vi "InstrumentsTree.vi"(1 "Type":string) -> (0 "Name":string)   [LabVIEW 2009]
uses:
  <userlib>/_OpenG.lib/array/array.llb/Conditional Auto-Indexing Tunnel (String)__ogtk.vi
panel:
  in  "Tree":string(tree)
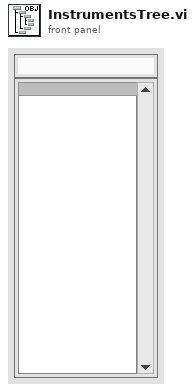
[diagram p1: front panel]
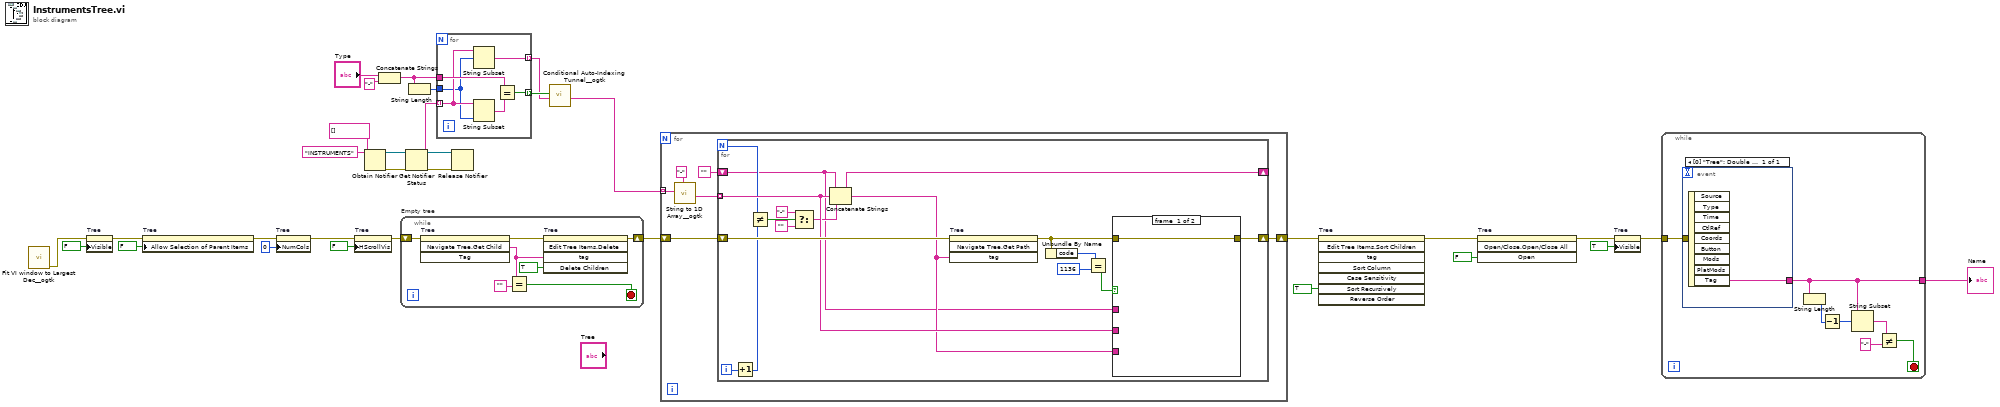
[diagram p0: block diagram]
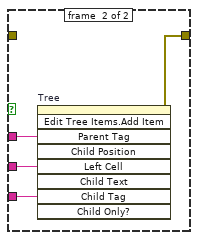
[diagram p2: hidden frame]
diagram:
  n1 = call <userlib>:"Fit VI window to Largest Dec__ogtk.vi"() -> ("error out"=w1:errorcluster)  [unwired: 3 in, 4 out]
  n2 = property on="Tree" class="Tree (strict)"(error in=w1, "Visible"=FALSE) -> (error out=w23:errorcluster)  [unwired: 1 in, 1 out]
  n3 = property on="Tree" class="Tree (strict)"(error in=w23, "Allow Selection of Parent Items"=FALSE) -> (error out=w28:errorcluster)  [unwired: 1 in, 1 out]
  n4 = property on="Tree" class="Tree (strict)"(error in=w28, "NumCols"=u32 0 ("Number of Columns")) -> (error out=w25:errorcluster)  [unwired: 1 in, 1 out]
  n5 = property on="Tree" class="Tree (strict)"(error in=w25, "HScrollVis"=FALSE ("Visible Items:Horizontal Scrollbar Visible")) -> (error out=w24:errorcluster)  [unwired: 1 in, 1 out]
  n6 = Obtain Notifier(name (unnamed)="INSTRUMENTS", notification data type=string[] [] ("Motor Names")) -> (notifier out=w13:refnum<notifier>, error out=w12:errorcluster)  [unwired: 2 in, 1 out]
  n7 = Concatenate Strings("Type", "-" ("string")) -> (w6:string)
  n8 = while "Empty tree" {
    shift-right: [w34] -> w32
    shift-left: w24 -> [w33]
    stop <- w36 stop-if-true
    n9 = invoke on="Tree" class="Tree (strict)" method="Navigate Tree.Get Child"(error in=w33) -> (error out=w35:errorcluster, "Navigate Tree:Get Child"=w38:string)  [unwired: 3 in, 2 out]
    n10 = Equal?(x=w38, y="") -> (x = y?=w36:bool)
    n11 = invoke on="Tree" class="Tree (strict)" method="Edit Tree Items.Delete"(error in=w35, "tag"=w38, "Delete Children"=TRUE ("Delete Children?")) -> (error out=w34:errorcluster)  [unwired: 2 in, 4 out]
  }
  n12 = Get Notifier Status(notifier=w13, error in (no error)=w12) -> (notifier out=w10:refnum<notifier>, current notification=w4:string[], error out=w11:errorcluster)  [unwired: 2 out]
  n13 = String Length(string=w6) -> (length=w9:i32)
  n14 = for {
    tunnel: w4 -> [w42] mode=indexing
    tunnel: w6 -> [w45]
    tunnel: w9 -> [w41]
    tunnel: [w43] -> w5 mode=indexing
    tunnel: [w40] -> w3 mode=indexing
    n15 = String Subset(string=w42, offset (0)=w41) -> (substring=w40:string)  [unwired: 1 out]
    n16 = String Subset(string=w42, length (rest)=w41) -> (substring=w44:string)  [unwired: 1 out]
    n17 = Equal?(x=w45, y=w44) -> (x = y?=w43:bool)
  }
  n18 = Release Notifier(notifier=w10, error in (no error)=w11) -> ()  [unwired: 4 out]
  n19 = call-poly <userlib>:"Conditional Auto-Indexing Tunnel__ogtk.vi"("Array in"=w3, "Elements to keep"=w5) -> ("Filtered Array out"=w2:string[])  [unwired: 5 out]
  n20 = for {
    tunnel: w2 -> [w48] mode=indexing
    shift-right: [w50] -> w31
    shift-left: w32 -> [w47]
    n21 = call <userlib>:"String to 1D Array__ogtk.vi"("delimiter (Tab)"="-", "string"=w48) -> ("Array of Strings"=w49:string[])  [unwired: 1 in, 8 out]
    n22 = for {
      N -> [w59]
      tunnel: w49 -> [w64] mode=indexing
      shift-right: [w63] -> w50
      shift-left: w47 -> [w67]
      shift-right: [w53] -> _
      shift-left: "" -> [w52]
      i -> [w60]
      n23 = Increment(x=w60) -> (x+1=w58:i32)
      n24 = Not Equal?(x=w59, y=w58) -> (x != y?=w57:bool)
      n25 = Select(t="-", s=w57, f="") -> (s? t:f=w54:string)
      n26 = Concatenate Strings(w52, w64, w54) -> (w53:string)
      n27 = invoke on="Tree" class="Tree (strict)" method="Navigate Tree.Get Path"(error in=w67, "tag"=w53) -> (error out=w61:errorcluster)  [unwired: 2 in, 3 out]
      n28 = Unbundle By Name(w61) -> ("code"=w66:i32)
      n29 = Equal?(x=w66, y=1136) -> (x = y?=w62:bool)
      n30 = case shown="True" w62 {
        tunnel: w64 -> [_ w72]
        tunnel: w53 -> [_ w71]
        tunnel: [w68 w70] -> w63
        tunnel: w61 -> [w68 _]
        tunnel: w52 -> [_ w69]
        frame #0 {
        }
        frame #1 {
          n31 = invoke on="Tree" class="Tree (strict)" method="Edit Tree Items.Add Item"("Parent Tag"=w69, "Left Cell"=w72, "Child Tag"=w71) -> (error out=w70:errorcluster)  [unwired: 6 in, 8 out]
        }
      }
    }
  }
  n32 = invoke on="Tree" class="Tree (strict)" method="Edit Tree Items.Sort Children"(error in=w31, "Sort Recursively"=TRUE ("Sort Recursively?")) -> (error out=w18:errorcluster)  [unwired: 6 in, 7 out]
  n33 = invoke on="Tree" class="Tree (strict)" method="Open/Close.Open/Close All"(error in=w18, "Open"=FALSE ("Open?")) -> (error out=w17:errorcluster)  [unwired: 2 in, 3 out]
  n34 = property on="Tree" class="Tree (strict)"(error in=w17, "Visible"=TRUE) -> (error out=w20:errorcluster)  [unwired: 1 in, 1 out]
  n35 = while {
    tunnel: w20 -> [w79]
    tunnel: [w78] -> w19
    stop <- w73 stop-if-true
    n36 = event shown="[0] \"Tree\": Double Click" {
      selector: _ -> [_]
      dyn-events: _ -> [_]
      timeout: _ -> [_]
      tunnel: w79 -> [_]
      tunnel: [w80] -> w78
      event [0] "Tree": Double Click {
        n37 = event-data() -> ("Tag"=w80:string)  [unwired: 9 out]
      }
    }
    n38 = String Length(string=w78) -> (length=w77:i32)
    n39 = Decrement(x=w77) -> (x-1=w76:i32)
    n40 = String Subset(string=w78, offset (0)=w76) -> (substring=w75:string)  [unwired: 1 out]
    n41 = Not Equal?(x=w75, y="-") -> (x != y?=w73:bool)
  }
  "Name" <- w19
